vi "Motic Find Camera.vi"(8 "error in (no error)":errorcluster) -> (0 "error out":errorcluster, 3 "camera out":i32)   [LabVIEW 2012, in "MoticApi.lvlib"]
doc: "MOTICAPI MUCam_Handle Motic_FindCamera();"
uses:
  MoticApi.lvlib
  MoticApi.dll
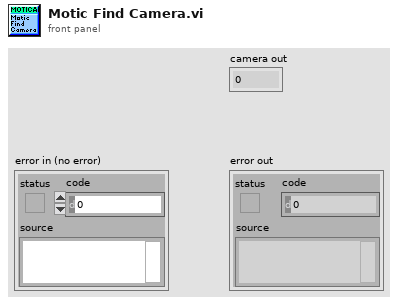
[diagram p1: front panel]
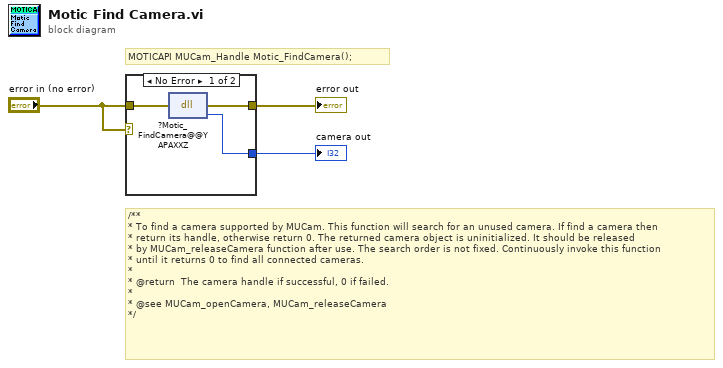
[diagram p0: block diagram]
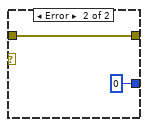
[diagram p2: hidden frame]
diagram:
  # "/**\n* To find a camera supported by MUCam. This function will search for an unused camera. If find a camera then\n* return its handle, otherwise return 0. The returned camera object is uninitialized. It should be released\n* by MUCam_releaseCamera function after use. The search order is not fixed. Continuously invoke this function\n* until it returns 0 to find all connected cameras.\n*\n* @return  The camera handle if successful, 0 if failed.\n*\n* @see MUCam_openCamera, MUCam_releaseCamera\n*/"
  # "MOTICAPI MUCam_Handle Motic_FindCamera();"
  n1 = case shown="No Error" "error in (no error)" {
    tunnel: [w6 0] -> w3
    tunnel: "error in (no error)" -> [w5 w8]
    tunnel: [w4 w8] -> w2
    frame No Error {
      n2 = dll-call lib="C:/Users/TTS-Digital/Desktop/MoticApi/MoticApi_git/MoticApi/MoticApi.*" fn="?Motic_FindCamera@@YAPAXXZ"(error in=w5) -> (error out=w4:errorcluster, w6:i32)  [unwired: 2 in, 1 out]
    }
    frame Error {
    }
  }
  "camera out" <- w3
  "error out" <- w2
